vi "RichToFlatrfcontrol_Response.vi"(5 "OutputClusterType":T1, 11 "InputCluster":T2) -> (3 "OutputCluster":T1)   [LabVIEW 2024, in "FlexCompute_grpc_client.lvlib"]
uses:
  rfcontrol_Response.ctl
  rfcontrol_Response_Flat.ctl
  FlexCompute_grpc_client.lvlib
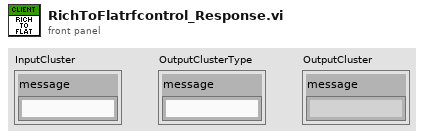
[diagram p1: front panel]
types:
  T1 = typedef "FlexCompute_grpc_client.lvlib/rfcontrol_Response_Flat.ctl" = cluster{"message":string}
  T2 = typedef "FlexCompute_grpc_client.lvlib/rfcontrol_Response.ctl" = cluster{"message":string}
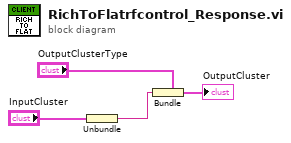
[diagram p0: block diagram]
diagram:
  n1 = Unbundle "Unbundle"("InputCluster") -> ("message"=w1:string)
  n2 = Bundle "Bundle"(cluster="OutputClusterType", "message"=w1) -> (→"OutputCluster":T1)
